vi "Periodic Tasks.vi"(8 "error in (no error)":errorcluster) -> ()   [LabVIEW 2014]
doc: "This VI runs in parallel to other tasks. It can contain as many user-defined periodic loops as you need. These can carry out PID or other sorts of timed response."
uses:
  <vilib>/Rock Robotics/SystemInterfaces/Typedef/FPGA_TypedefAnalogModule.ctl
  <vilib>/Rock Robotics/SystemInterfaces/AI/FPGA_AIChannel.ctl
  <vilib>/Rock Robotics/SystemInterfaces/Typedef/FPGA_TypedefDigitalModule.ctl
  <vilib>/Rock Robotics/SystemInterfaces/i2clib/i2c_bus.ctl
  <vilib>/Rock Robotics/WPI/Joystick/WPI_JoystickGetSetRefNum.vi
  <vilib>/Rock Robotics/WPI/RobotDrive/WPI_RobotDriveGetSetRefNum.vi
  <vilib>/Rock Robotics/Network Tables/SD Read Number.vi
  <vilib>/Rock Robotics/Network Tables/SD Write Numeric Array.vi
  <vilib>/Rock Robotics/Network Tables/SD Write Number.vi
panel:
  out "Data Out":u8[](array[numeric])
  in  "I2CBytesToRead":u8=10
  out "LED_Off":u32(colorbox)=16775840
  in  "Position Speed":u32(slide)=20 scale=5.0..2000.0
  out "LED_On":u32(colorbox)=65282
  out "LED Position":u8(slide)=7 scale=0.0..30.0
  in  "Brightness":u8(slide)=255 scale=0.0..255.0
  out "error out":errorcluster
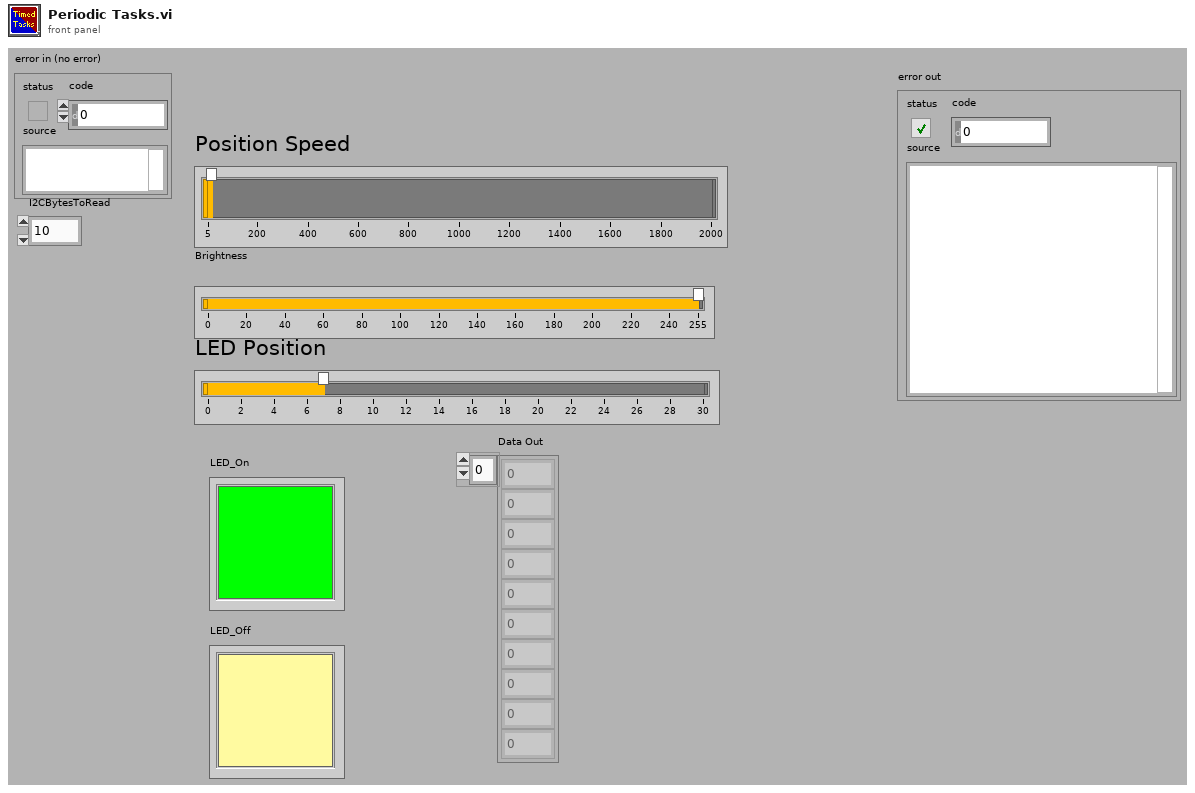
[diagram p1: front panel]
types:
  T1 = typedef "i2c_bus.ctl" = enum16{"I2C On-Board", "I2C MXP", "Invalid"}
  T2 = typedef "FPGA_TypedefDigitalModule.ctl" = enum16{"Controller 1"}
  T3 = typedef "FPGA_AIChannel.ctl" = enum8{"AI 0", "AI 1", "AI 2", "AI 3", "AI MXP 0", "AI MXP 1", "AI MXP 2", "AI MXP 3", "Invalid"}
  T4 = typedef "FPGA_TypedefAnalogModule.ctl" = enum16{"Controller 1"}
  T5 = typedef "WPI_I2CDevRef.ctl" = cluster{"DevStatus":errorcluster, "Controller":T2, "Device Address":u8, "Handle":i32, "I2C Bus":T1}
  T6 = typedef "WPI_AnalogChannelDevRef.ctl" = cluster{"DevStatus":errorcluster, "Controller":T4, "Analog Channel":T3}
  T7 = typedef "WPI_JoystickDevRef.ctl" = cluster{"Device":T8}
  T8 = typedef "WPI_JoystickDeviceEnum.ctl" = enum16{"USB 0", "USB 1", "USB 2", "USB 3", "USB 4", "USB 5"}
  T9 = typedef "WPI_RobotDriveDevRef.ctl" = cluster{"DevStatus":errorcluster, "Motors[]":T10[], "Square Inputs":bool, "Max Output":dbl}
  T10 = typedef "WPI_MotorControlDeviceRef.ctl" = cluster{"DeviceStatus":errorcluster, "Type":T11, "PWM":cluster{"Controller":T2, "PWM Channel":T12, "DeadBand":T13}, "CAN":cluster{"Device Number":u8, "Control Mode":T14, "Semaphore":T15, "Max Vout":dbl, "TalonSRX Control Mode":T16}, "Invert":bool, "TransformRef":T17, "InvTransformRef":T17}
  T11 = typedef "WPI_MotorControlType.ctl" = enum16{"PWM", "CAN", "CANTalonSRX"}
  T12 = typedef "FPGA_DIOPWMChannel.ctl" = enum8{"PWM 0", "PWM 1", "PWM 2", "PWM 3", "PWM 4", "PWM 5", "PWM 6", "PWM 7", "PWM 8", "PWM 9", "PWM MXP 0", "PWM MXP 1", "PWM MXP 2", "PWM MXP 3", "PWM MXP 4", "PWM MXP 5", "PWM MXP 6", "PWM MXP 7", "PWM MXP 8", "PWM MXP 9", "Invalid"}
  T13 = typedef "WPI_PWMDeadband.ctl" = cluster{"Name":string, "maxPositivePwm":i32, "minPositivePwm":i32, "centerPwm":i32, "maxNegativePwm":i32, "minNegativePwm":i32, "angularRange":u16}
  T14 = typedef "WPI_CANJaguar_ControlMode.ctl" = enum8{"Percent VBus", "Current", "Speed", "Position", "Voltage"}
  T15 = typedef "Semaphore RefNum" = refnum<k1>
  T16 = typedef "WPI_CANTalonSRX_APIControlMode.ctl" = enum8{"Percent VBus", "Speed", "Position", "Slave", "Unchanged / Invalid"}
  T17 = typedef "WPI_PWMTransform_ConPane.ctl" = refnum<vi>
  T18 = cluster{"JoystickDevRef":T7, "RobotDriveDevRef":T9}
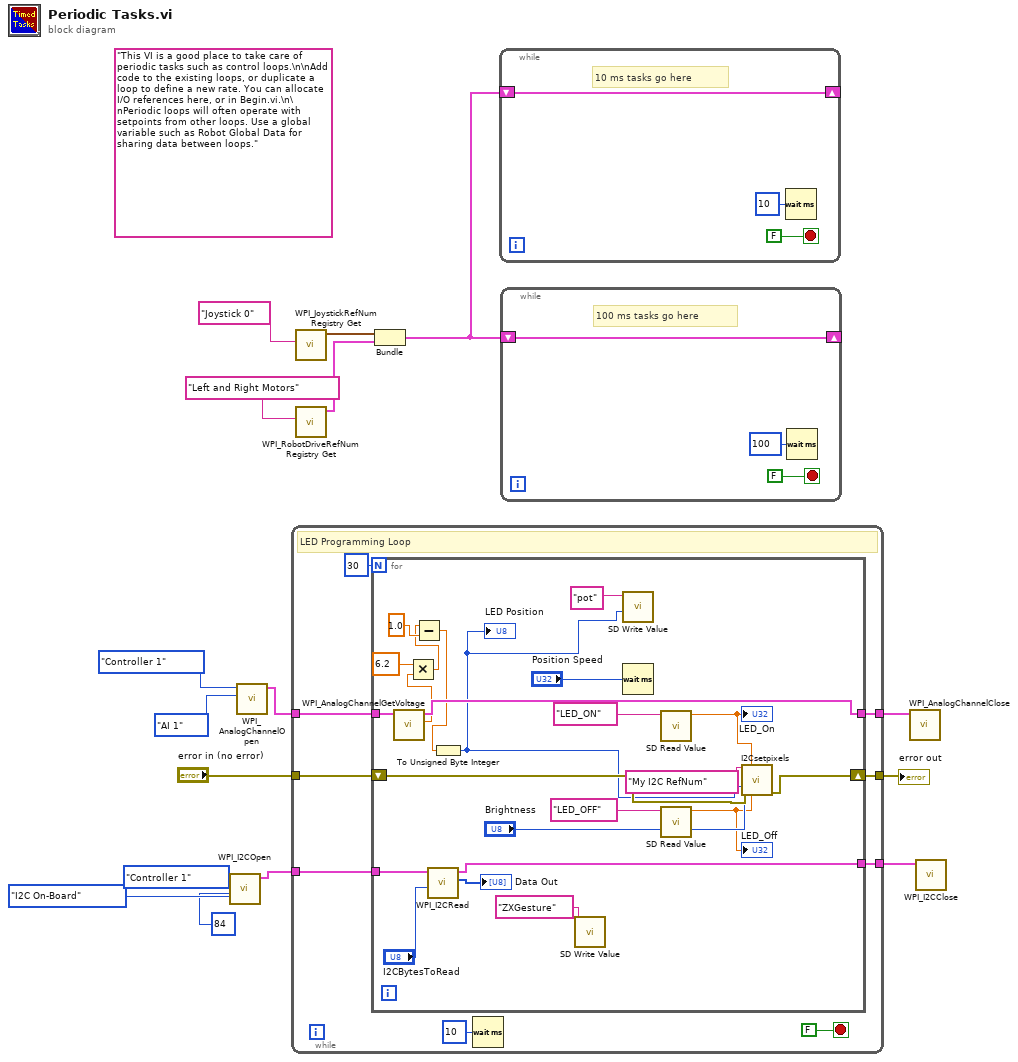
[diagram p0: block diagram]
diagram:
  (unwired) "This VI is a good place to take care of periodic tasks such as control loops.\n\nAdd code to the existing loops, or duplicate a loop to define a new rate. You can allocate I/O references here, or in Begin.vi.\n\nPeriodic loops will often operate with setpoints from other loops. Use a global variable such as Robot Global Data for sharing data between loops."
  n1 = call <vilib>:"WPI_I2COpen.vi"("Device Address"=u8 84, "I2C Bus"=i2c_bus."I2C On-Board", "Controller"=FPGA_TypedefDigitalModule."Controller 1") -> ("I2CDevRef"=w5:T5)  [unwired: 7 in, 1 out]
  n2 = call <vilib>:"WPI_AnalogChannelOpen.vi"("Analog Channel"=FPGA_AIChannel."AI 1", "Controller"=FPGA_TypedefAnalogModule."Controller 1") -> ("AIDeviceRef"=w7:T6)  [unwired: 8 in, 1 out]
  n3 = while {
    tunnel: "error in (no error)" -> [w24]
    tunnel: [w21] -> w10
    tunnel: w7 -> [w20]
    tunnel: [w19] -> w6
    tunnel: w5 -> [w18]
    tunnel: [w17] -> w4
    stop <- FALSE stop-if-true
    # "LED Programming Loop"
    n4 = for {
      N: 30 -> [_]
      shift-right: [w47] -> w21
      shift-left: w24 -> [w48]
      tunnel: w20 -> [w43]
      tunnel: [w42] -> w19
      tunnel: w18 -> [w30]
      tunnel: [w29] -> w17
      n5 = call <vilib>:"WPI_AnalogChannelGetVoltage.vi"("AIDeviceRef"=w43) -> ("Voltage"=w40:dbl, "AIDeviceRef"=w42:T6)  [unwired: 8 in, 1 out]
      n6 = Multiply(x=6.2, y=w40) -> (x*y=w38:dbl)
      n7 = Subtract(x=w38, y=1.0 ("x")) -> (x-y=w33:dbl)
      n8 = call <vilib>:"WPI_I2CRead.vi"("I2CBytesToRead"="I2CBytesToRead", "I2CDevRef"=w30) -> ("Data Out"=→"Data Out":u8[], "I2CDevRef"=w29:T5)  [unwired: 7 in, 1 out]
      n9 = To Unsigned Byte Integer(number=w33) -> (unsigned 8bit integer=w31:u8)
      "LED Position" <- w31
      n10 = call-poly <vilib>:"SD Write Value.vi"("Name"="ZXGesture") -> ()  [unwired: 9 in, 2 out]
      n11 = call-poly <vilib>:"SD Write Value.vi"("Numeric"=w31, "Name"="pot") -> ()  [unwired: 8 in, 2 out]
      n12 = Wait (ms)(milliseconds to wait="Position Speed") -> ()  [unwired: 1 out]
      n13 = call-poly <vilib>:"SD Read Value.vi"("Name"="LED_ON") -> ("Numeric"=w36:dbl)  [unwired: 8 in, 2 out]
      "LED_On" <- w36
      n14 = call-poly <vilib>:"SD Read Value.vi"("Name"="LED_OFF") -> ("Numeric"=w34:dbl)  [unwired: 8 in, 2 out]
      "LED_Off" <- w34
      n15 = call "I2Csetpixels.vi"("I2C Reference In"="My I2C RefNum" ("refnum name"), "Color Box - On"=w36, "Brightness (0-255)"="Brightness", "LED Position"=w31, "Error In"=w48, "Color Box - Off"=w34) -> ("Error Out"=w47:errorcluster)  [unwired: 8 in, 1 out]
    }
    n16 = Wait (ms)(milliseconds to wait=u32 10) -> ()  [unwired: 1 out]
  }
  "error out" <- w10
  n17 = call <vilib>:"WPI_JoystickRefNum Registry Get.vi"("refnum name"="Joystick 0") -> ("JoystickDevRef"=w14:T7)  [unwired: 1 in, 9 out]
  n18 = call <vilib>:"WPI_RobotDriveRefNum Registry Get.vi"("refnum name"="Left and Right Motors") -> ("RobotDriveDevRef"=w13:T9)  [unwired: 1 in, 9 out]
  n19 = Bundle("JoystickDevRef"=w14, "RobotDriveDevRef"=w13) -> (w12:T18)  [unwired: 1 out]
  n20 = while {
    shift-right: [w49] -> _
    shift-left: w12 -> [w49]
    stop <- FALSE stop-if-true
    # "10 ms tasks go here"
    n21 = Wait (ms)(milliseconds to wait=u32 10) -> ()  [unwired: 1 out]
  }
  n22 = while {
    shift-right: [w52] -> _
    shift-left: w12 -> [w52]
    stop <- FALSE stop-if-true
    # "100 ms tasks go here"
    n23 = Wait (ms)(milliseconds to wait=u32 100) -> ()  [unwired: 1 out]
  }
  n24 = call <vilib>:"WPI_AnalogChannelClose.vi"("AIDeviceRef"=w6) -> ()  [unwired: 10 in, 1 out]
  n25 = call <vilib>:"WPI_I2CClose.vi"("I2CDevRef"=w4) -> ()  [unwired: 10 in, 1 out]
